vi "OpenTstFileRef.vi"(8 "ErrorArray":errorcluster[](array[cluster])) -> (0 "ErrorArray":errorcluster[](array[cluster]), 3 "refnum":T1)   [LabVIEW 2017, in "Framework.lvlib"]
uses:
  Framework.lvlib
  <vilib>/Utility/config.llb/Config Data RefNum.ctl
  Config_class/Config.lvclass/Config.ctl
  Config_class/Accessors/Read PARTF Root Directory.vi
  <vilib>/Utility/error.llb/Error Cluster From Error Code.vi
  <vilib>/ErrorRing/Error Ring.xnode
  Config_class/Config.lvclass
  <vilib>/Utility/config.llb/NI_LVConfig.lvlib
  <userlib>/NIST/NISTErrorLib/NISTErrorLib.lvlib
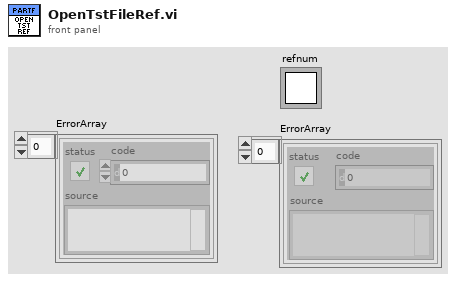
[diagram p1: front panel]
types:
  T1 = typedef "NI_LVConfig.lvlib/Config Data RefNum.ctl" = refnum<k1>
  T2 = typedef "Framework.lvlib/clFrontPanelControlRefs.ctl" = cluster{"TestFilePathRef":refnum<vi>, "BusNumberRef":refnum<vi>, "NumberOfBusesRef":refnum<vi>, "EvtTypeRef":refnum<vi>, "EvtParamsRef":refnum<vi>, "EvtConfigRef":refnum<vi>, "StartTimeRef":refnum<vi>, "EndTimeRef":refnum<vi>, "PmuImpairTypeRef":refnum<vi>, "PmuImpairParamsRef":refnum<vi>, "NetImpairParamsRef":refnum<vi>, "FlagImpairTypeRef":refnum<vi>, "FlagImpairParamsRef":refnum<vi>, "NetImpairTypeRef":refnum<vi>, "OutputFileType":refnum<vi>, "PmuImpairConfigRef":refnum<vi>, "AppTypeRef":refnum<vi>, "ScriptPathRef":refnum<vi>, "ShowPanels?":refnum<vi>}
  T3 = typedef "Framework.lvlib/Config.lvclass/RootDir.ctl" = cluster{"pathRootDir":path, "btnOutPath":bool, "OutDir":string, "btnOpenOutputDir":bool, "ScriptDir":string, "btnOpenScriptDir":bool, "TestDir":string, "btnOpenTestDir":bool}
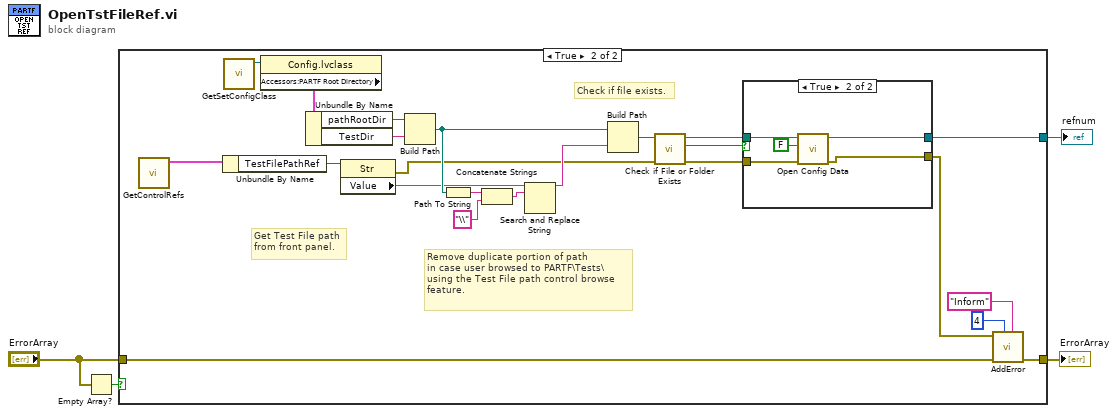
[diagram p0: block diagram]
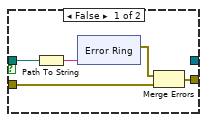
[diagram p3: hidden frame]
diagram:
  n1 = Empty Array?(array="ErrorArray") -> (empty?=w2:bool)
  n2 = case shown="True" w2 {
    tunnel: [_ w13] -> w4
    tunnel: "ErrorArray" -> [w5 w12]
    tunnel: [w5 w11] -> w3
    frame False {
    }
    frame True {
      # "Check if file exists."
      # "Get Test File path\nfrom front panel."
      # "Remove duplicate portion of path\nin case user browsed to PARTF\\Tests\\\nusing the Test File path control browse\nfeature."
      n3 = call "GetControlRefs.vi"() -> ("clControlRefs Out"=w7:T2)  [unwired: 11 in]
      n4 = Unbundle By Name(w7) -> ("TestFilePathRef"=w18:refnum<vi>)
      n5 = call "GetSetConfigClass.vi"() -> ("Ref out"=w25:refnum<class "Config.lvclass">)  [unwired: 11 in]
      n6 = property class="Config.lvclass"(reference=w25) -> ("Accessors:PARTF Root Directory"=w26:T3)  [unwired: 1 in, 2 out]
      n7 = Unbundle By Name(w26) -> ("pathRootDir"=w27:path, "TestDir"=w28:string)
      n8 = property class="Str"(reference=w18) -> (error out=w19:errorcluster, "Value"=w6:string)  [unwired: 1 in, 1 out]
      n9 = Build Path(base path=w27, name or relative path=w28) -> (appended path=w23:path)
      n10 = Path To String(path=w23) -> (string=w20:string)
      n11 = Concatenate Strings(w20, "\\" ("string")) -> (w21:string)
      n12 = Search and Replace String(input string=w6, search string=w21) -> (result string=w24:string)  [unwired: 6 in, 3 out]
      n13 = Build Path(base path=w23, name or relative path=w24) -> (appended path=w14:path)
      n14 = call <vilib>:"Check if File or Folder Exists.vi"("error in (no error)"=w19, "path"=w14) -> ("error out"=w17:errorcluster, "file or folder exists?"=w15:bool, "dup path"=w16:path)  [unwired: 7 in]
      n15 = case shown="True" w15 {
        tunnel: w17 -> [w30 w43]
        tunnel: w16 -> [w32 w45]
        tunnel: [w29 w42] -> w10
        tunnel: [_ w41] -> w13
        frame False {
          n16 = Path To String(path=w32) -> (string=w33:string)
          n17 = xnode "Error Ring"("parameter 0"=w33) -> ("error out"=w31:errorcluster)
          n18 = Merge Errors(w31, w30) -> (w29:errorcluster)
        }
        frame True {
          n19 = call <vilib>:"Open Config Data.vi"("error in (no error)"=w43, "create file if necessary (T)"=FALSE, "configuration file path"=w45) -> ("error out"=w42:errorcluster, "refnum"=w41:T1)  [unwired: 6 in, 1 out]
        }
      }
      n20 = call <userlib>:"AddError.vi"("Severity"="Inform", "Priority"=u8 4, "ErrorArray"=w12, "error in (no error)"=w10) -> ("ErrorArray"=w11:errorcluster[])  [unwired: 6 in, 1 out]
    }
  }
  "refnum" <- w4
  "ErrorArray" <- w3
